vi "Autofocus Step.vi"(8 "error in (no error)":errorcluster, 10 "Frame Number\n(starts with 1)":i32, 11 "Stage Controller in":refnum<class "Stage Controller.lvclass">) -> (0 "error out":errorcluster, 3 "Stage Controller out":refnum<class "Stage Controller.lvclass">)   [LabVIEW 2018, in "Stage Controller.lvlib" / "Stage Controller.lvclass"]
uses:
  Stage Controller.lvclass
  Stage Controller.lvclass/Stage Controller.ctl
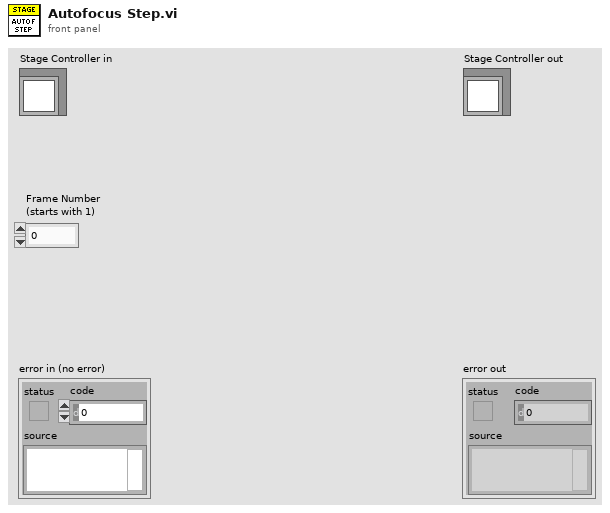
[diagram p1: front panel]
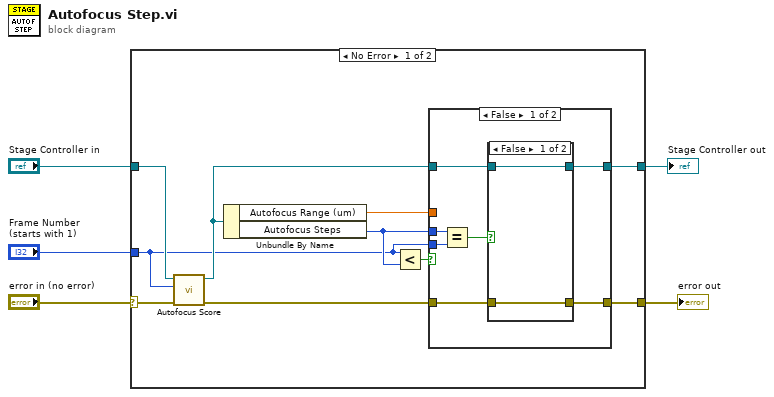
[diagram p0: block diagram]
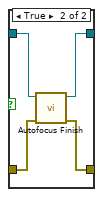
[diagram p2: hidden frame]
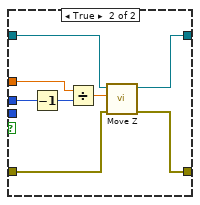
[diagram p3: hidden frame]
diagram:
  n1 = case shown="No Error" "error in (no error)" {
    selector: "error in (no error)" -> [w10 w38]
    tunnel: [w11 w38] -> w4
    tunnel: [w12 w37] -> w1
    tunnel: "Stage Controller in" -> [w8 w37]
    tunnel: "Frame Number\n(starts with 1)" -> [w6 _]
    frame No Error {
      n2 = call-dynamic "Autofocus Score.vi"("error in (no error)"=w10, "Frame Index"=w6, "Stage Controller in"=w8) -> ("error out"=w9:errorcluster, "Stage Controller out"=w7:refnum<class "Stage Controller.lvclass">)  [unwired: 7 in]
      n3 = Unbundle By Name(w7) -> ("Autofocus Range (um)"=w14:dbl, "Autofocus Steps"=w15:i32)
      n4 = Less?(x=w6, y=w15) -> (x < y?=w13:bool)
      n5 = case shown="False" w13 {
        tunnel: w7 -> [w22 w36]
        tunnel: [w20 w35] -> w12
        tunnel: w9 -> [w21 w34]
        tunnel: [w19 w33] -> w11
        tunnel: w15 -> [w18 w29]
        tunnel: w14 -> [_ w32]
        tunnel: w6 -> [w17 _]
        frame False {
          n6 = Equal?(x=w18, y=w17) -> (x = y?=w16:bool)
          n7 = case shown="False" w16 {
            tunnel: w22 -> [w23 w28]
            tunnel: w21 -> [w24 w27]
            tunnel: [w23 w26] -> w20
            tunnel: [w24 w25] -> w19
            frame False {
            }
            frame True {
              n8 = call-dynamic "Autofocus Finish.vi"("error in (no error)"=w27, "Stage Controller in"=w28) -> ("error out"=w25:errorcluster, "Stage Controller out"=w26:refnum<class "Stage Controller.lvclass">)  [unwired: 8 in]
            }
          }
        }
        frame True {
          n9 = Decrement(x=w29) -> (x-1=w30:i32)
          n10 = Divide(x=w32, y=w30) -> (x/y=w31:dbl)
          n11 = call-dynamic "Move Z.vi"("error in (no error)"=w34, "Delta (um)"=w31, "Stage Controller in"=w36) -> ("error out"=w33:errorcluster, "Stage Controller out"=w35:refnum<class "Stage Controller.lvclass">)  [unwired: 7 in]
        }
      }
    }
    frame Error {
    }
  }
  "error out" <- w4
  "Stage Controller out" <- w1
